vi "Rings.vi"(8 "error in (no error)":errorcluster, 11 "Rings":i32) -> (0 "error out":errorcluster)   [LabVIEW 2017]
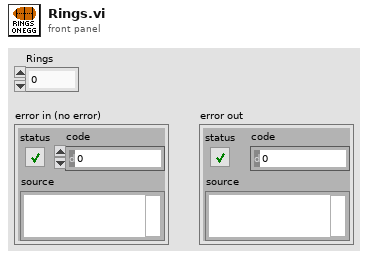
[diagram p1: front panel]
types:
  T1 = cluster{"MS1 (A/DIO1 (Pin 13))":bool, "MS2 (A/DIO2 (Pin 15))":bool, "MS3 (A/DIO3 (Pin 17))":bool}
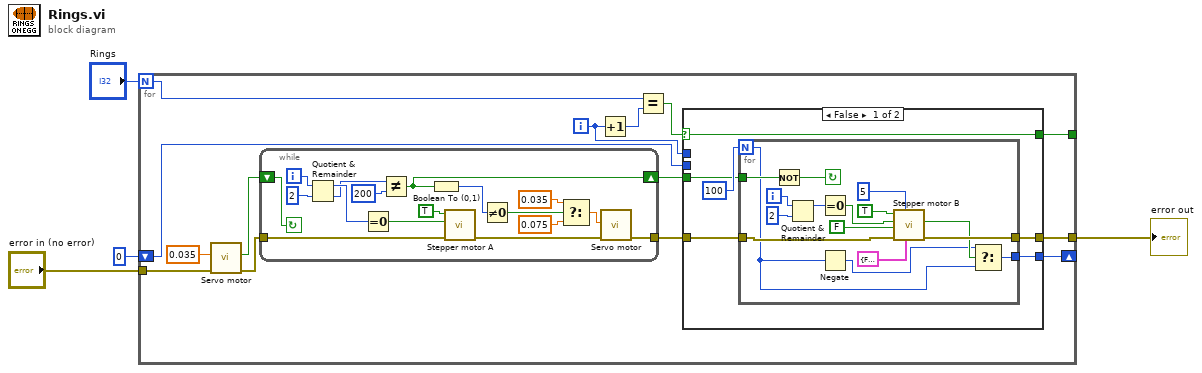
[diagram p0: block diagram]
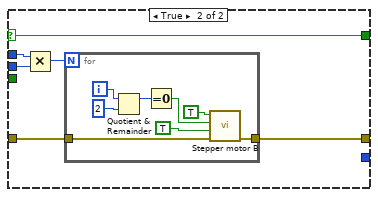
[diagram p2: hidden frame]
diagram:
  n1 = for {
    N: "Rings" -> [w10]
    tunnel: [w18] -> w1
    shift-right: [w9] -> _
    shift-left: 0 -> [w8]
    tunnel: "error in (no error)" -> [w6]
    tunnel: [w5] -> _
    i -> [w7]
    n2 = call "Servo motor.vi"("error in (no error)"=w6, "Duty Cycle"=0.035) -> ("error out"=w16:errorcluster, "Drop?"=w17:bool)  [unwired: 8 in]
    n3 = while {
      shift-right: [w63] -> w13
      shift-left: w17 -> [w64]
      tunnel: [w55] -> w15
      tunnel: w16 -> [w62]
      i -> [w70]
      stop <- w64 continue-if-true
      n4 = Quotient & Remainder(x=w70, y=2) -> (x-y*floor(x/y)=w68:i32, floor(x/y)=w66:i32)
      n5 = Equal To 0?(x=w68) -> (x = 0?=w67:bool)
      n6 = Not Equal?(x=w66, y=200) -> (x != y?=w63:bool)
      n7 = Boolean To (0,1)(Boolean=w63) -> (0, 1=w61:i16)
      n8 = call "Stepper motor A.vi"("error in (no error)"=w62, "Step (C/DIO3 (DIO3))"=w67, "Enable (C/DIO2 (DIO2))"=TRUE) -> ("error out"=w56:errorcluster)  [unwired: 8 in]
      n9 = Not Equal To 0?(x=w61) -> (x != 0?=w60:bool)
      n10 = Select(t=0.035, s=w60, f=0.075) -> (s? t:f=w59:dbl)
      n11 = call "Servo motor.vi"("error in (no error)"=w56, "Duty Cycle"=w59) -> ("error out"=w55:errorcluster)  [unwired: 8 in, 1 out]
    }
    n12 = Increment(x=w7) -> (x+1=w12:i32)
    n13 = Equal?(x=w10, y=w12) -> (x = y?=w11:bool)
    n14 = case shown="False" w11 {
      selector: w11 -> [w19 w41]
      tunnel: [w24 w45] -> w18
      tunnel: w15 -> [w22 w46]
      tunnel: w13 -> [w21 _]
      tunnel: w7 -> [_ w44]
      tunnel: [w20 _] -> w9
      tunnel: w8 -> [_ w42]
      tunnel: [w19 w41] -> w5
      frame False {
        n15 = for {
          N: 100 ("Numeric Control") -> [w26]
          tunnel: w22 -> [w34]
          tunnel: [w33] -> w24
          tunnel: w21 -> [w30]
          tunnel: [w25] -> w20
          i -> [w36]
          stop <- w35 continue-if-true
          n16 = Not(x=w30) -> (.not. x?=w35:bool)
          n17 = Quotient & Remainder(x=w36, y=2) -> (x-y*floor(x/y)=w38:i32)  [unwired: 1 out]
          n18 = Equal To 0?(x=w38) -> (x = 0?=w37:bool)
          n19 = Negate(x=w26) -> (-x=w27:i32)
          n20 = call "Stepper motor B.vi"("Microstepping"=T1 {"MS1 (A/DIO1 (Pin 13))"=FALSE, "MS2 (A/DIO2 (Pin 15))"=FALSE, "MS3 (A/DIO3 (Pin 17))"=FALSE}, "Speed"=u32 5, "error in (no error)"=w34, "Direction (A/DIO5 (Pin 21))"=FALSE, "Step (A/DIO4 (Pin 19))"=w37, "Enable (A/DIO0 (Pin 11))"=TRUE) -> ("error out"=w33:errorcluster, "Direction"=w28:bool)  [unwired: 4 in]
          n21 = Select(t=w27, s=w28, f=w26) -> (s? t:f=w25:i32)
        }
      }
      frame True {
        n22 = Multiply(x=w44, y=w42) -> (x*y=w43:i32)
        n23 = for {
          N: w43 -> [_]
          tunnel: w46 -> [w53]
          tunnel: [w52] -> w45
          i -> [w51]
          n24 = Quotient & Remainder(x=w51, y=2) -> (x-y*floor(x/y)=w49:i32)  [unwired: 1 out]
          n25 = Equal To 0?(x=w49) -> (x = 0?=w48:bool)
          n26 = call "Stepper motor B.vi"("error in (no error)"=w53, "Direction (A/DIO5 (Pin 21))"=TRUE, "Step (A/DIO4 (Pin 19))"=w48, "Enable (A/DIO0 (Pin 11))"=TRUE) -> ("error out"=w52:errorcluster)  [unwired: 6 in, 1 out]
        }
      }
    }
  }
  "error out" <- w1
